vi "Autonomous Independent.vi"() -> ()   [LabVIEW 2012]
doc: "This VI is called when autonomous begins, and will automatically be terminated when autonomous ends. You can carry out timed or sensor driven robot movement independently without needing to return to the caller."
uses:
  Robot Global Data.vi
  <vilib>/Rock Robotics/WPI/RobotDrive/WPI_RobotDriveGetSetRefNum.vi
  <vilib>/Rock Robotics/WPI/Joystick/WPI_JoystickGetSetRefNum.vi
panel:
  in  "Turn Amount":i32=90
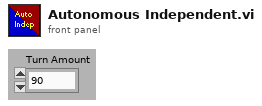
[diagram p1: front panel]
types:
  T1 = typedef "WPI_JoystickDevRef.ctl" = cluster{"Device":T2}
  T2 = typedef "WPI_JoystickDeviceEnum.ctl" = enum16{"USB 1", "USB 2", "USB 3", "USB 4", "Kinect 1", "Kinect 2"}
  T3 = cluster{"axis 1 (x)":dbl, "axis 2 (y)":dbl, "axis 3 (throttle)":dbl, "axis 4":dbl, "axis 5":dbl, "axis 6":dbl}
  T4 = typedef "WPI_RobotDriveDevRef.ctl" = cluster{"DevStatus":errorcluster, "Motors[]":T5[], "Square Inputs":bool, "Max Output":dbl, "Isochronous":bool}
  T5 = typedef "WPI_MotorControlDeviceRef.ctl" = cluster{"DeviceStatus":errorcluster, "Type":enum16{"PWM", "CAN"}, "PWM":cluster{"Digital Module":T6, "PWM Channel":T7, "DeadBand":T8}, "CAN":cluster{"Device Number":u8, "Control Mode":T9, "Semaphore":T10, "Max Vout":dbl}, "Invert":bool, "TransformRef":T11, "InvTransformRef":T11}
  T6 = typedef "FPGA_TypedefDigitalModule.ctl" = enum16{"Digital Module 1", "Digital Module 2"}
  T7 = typedef "FPGA_DIOPWMChannel.ctl" = enum8{"PWM 1", "PWM 2", "PWM 3", "PWM 4", "PWM 5", "PWM 6", "PWM 7", "PWM 8", "PWM 9", "PWM 10", "Invalid"}
  T8 = typedef "WPI_PWMDeadband.ctl" = cluster{"Name":string, "maxPositivePwm":i32, "minPositivePwm":i32, "centerPwm":i32, "maxNegativePwm":i32, "minNegativePwm":i32, "angularRange":u16}
  T9 = typedef "WPI_CANJaguar_ControlMode.ctl" = enum8{"Percent VBus", "Current", "Speed", "Position", "Voltage"}
  T10 = typedef "Semaphore RefNum" = refnum<k1>
  T11 = typedef "WPI_PWMTransform_ConPane.ctl" = refnum<vi>
  T12 = typedef "WPI_GyroDevRef.ctl" = cluster{"DevStatus":errorcluster, "Analog Module":T13, "Analog Channel":T14, "Offset":dbl, "Gain (VoltsPerDegree/Second)":dbl}
  T13 = typedef "FPGA_TypedefAnalogModule.ctl" = enum16{"Analog Module 1", "Analog Module 2"}
  T14 = typedef "FPGA_AIChannel.ctl" = enum8{"AI 1", "AI 2", "AI 3", "AI 4", "AI 5", "AI 6", "AI 7", "AI 8", "Invalid"}
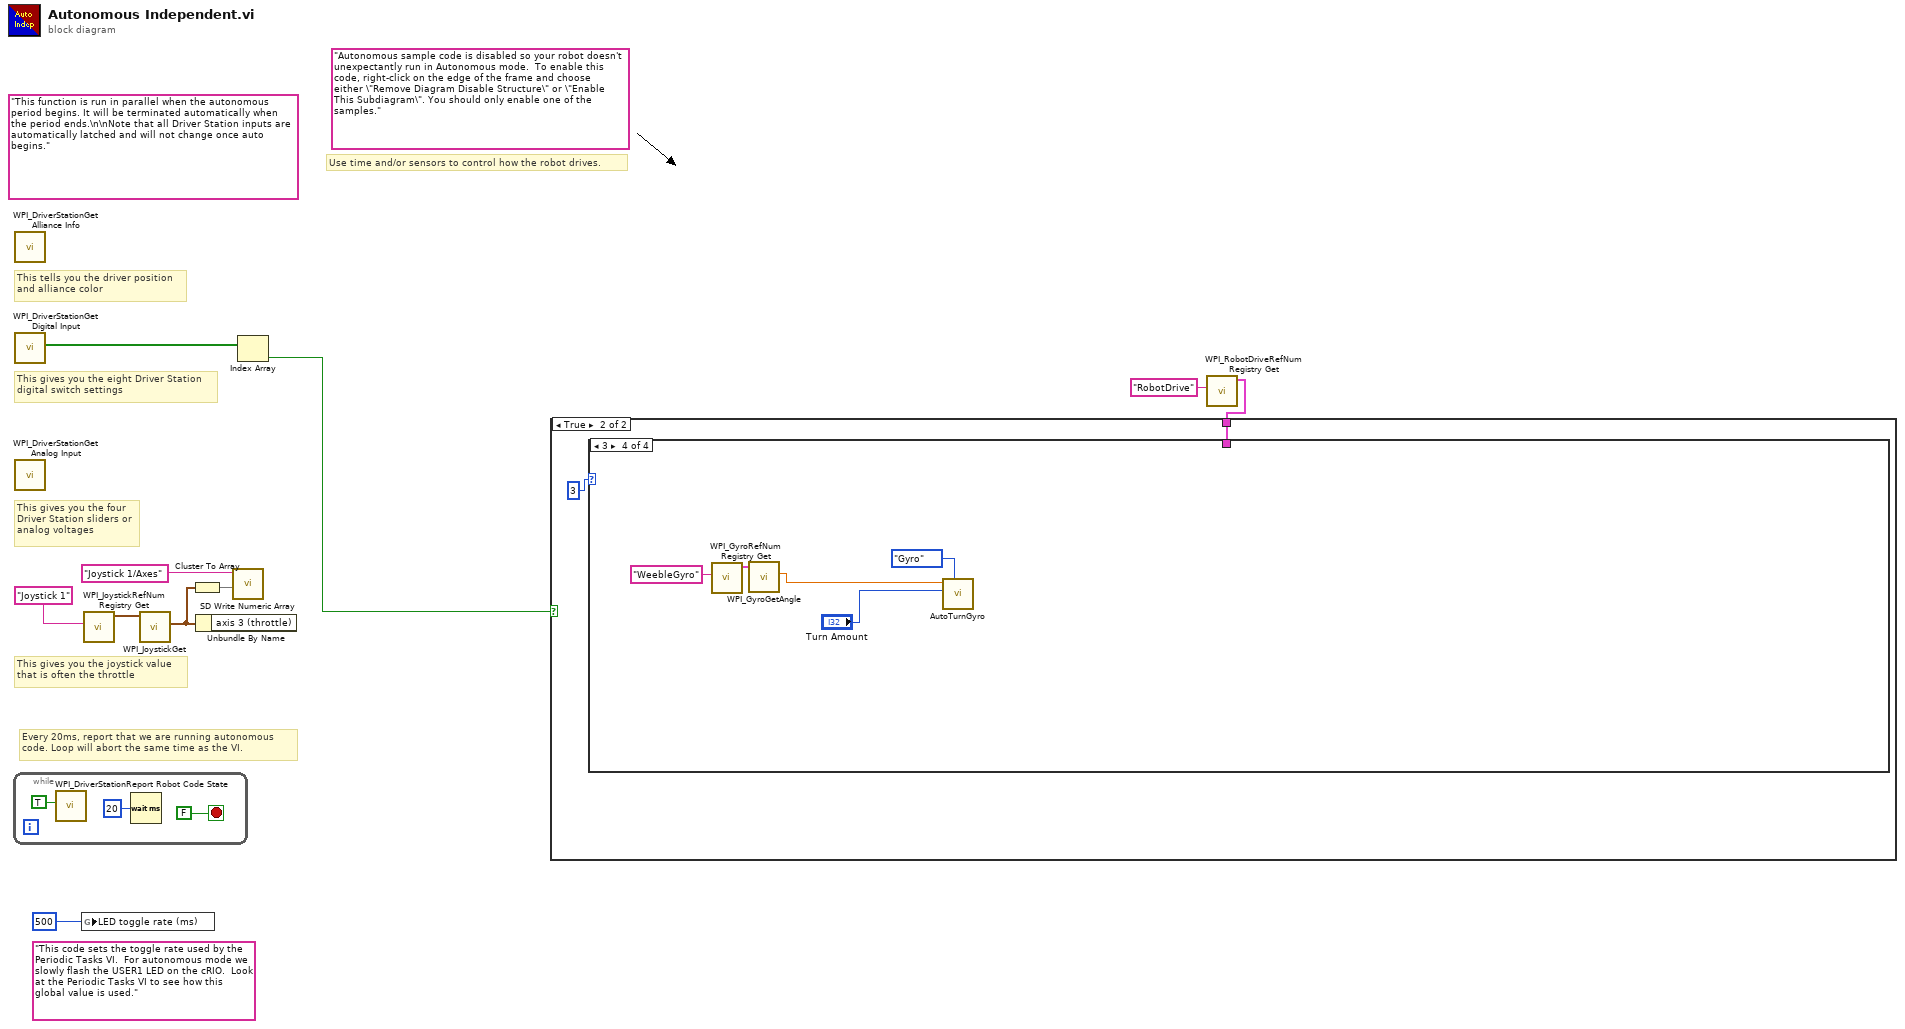
[diagram p0: block diagram]
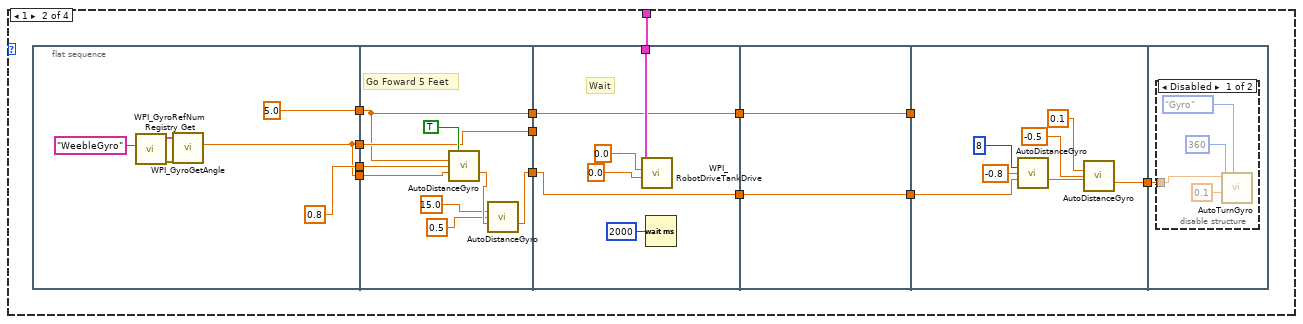
[diagram p4: hidden frame]
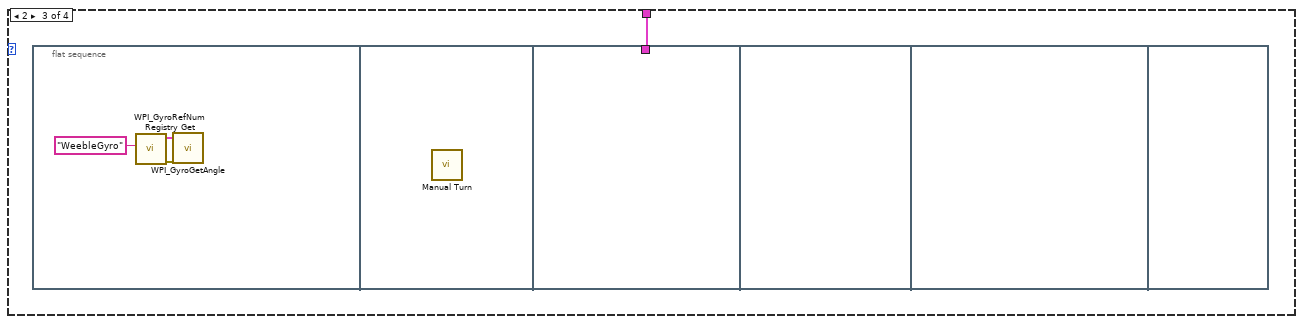
[diagram p6: hidden frame]
diagram:
  (unwired) "This code sets the toggle rate used by the Periodic Tasks VI.  For autonomous mode we slowly flash the USER1 LED on the cRIO.  Look at the Periodic Tasks VI to see how this global value is used."
  (unwired) "Autonomous sample code is disabled so your robot doesn't unexpectantly run in Autonomous mode.  To enable this code, right-click on the edge of the frame and choose either \"Remove Diagram Disable Structure\" or \"Enable This Subdiagram\". You should only enable one of the samples."
  (unwired) "This function is run in parallel when the autonomous period begins. It will be terminated automatically when the period ends.\n\nNote that all Driver Station inputs are automatically latched and will not change once auto begins."
  # "Every 20ms, report that we are running autonomous\ncode. Loop will abort the same time as the VI."
  # "This gives you the joystick value\nthat is often the throttle"
  # "Use time and/or sensors to control how the robot drives."
  # "This tells you the driver position\nand alliance color"
  # "This gives you the eight Driver Station\ndigital switch settings"
  # "This gives you the four\nDriver Station sliders or\nanalog voltages"
  n1 = while {
    stop <- FALSE stop-if-true
    n2 = call <vilib>:"WPI_DriverStationReport Robot Code State.vi"("Autonomous"=TRUE) -> ()  [unwired: 10 in, 1 out]
    n3 = Wait (ms)(milliseconds to wait=u32 20) -> ()  [unwired: 1 out]
  }
  n4 = call <vilib>:"WPI_DriverStationGet Alliance Info.vi"() -> ()  [unwired: 12 out]
  n5 = call <vilib>:"WPI_DriverStationGet Digital Input.vi"() -> ("Driver Station Digital Input (1-8)"=w10:bool[])  [unwired: 11 out]
  n6 = call <vilib>:"WPI_DriverStationGet Analog Input.vi"() -> ()  [unwired: 12 out]
  n7 = global write "Robot Global Data.vi" "LED toggle rate (ms)"(u32 500 ("LED ms toggle rate")) -> ()
  n8 = call <vilib>:"WPI_JoystickRefNum Registry Get.vi"("refnum name"="Joystick 1") -> ("JoystickDevRef"=w8:T1)  [unwired: 1 in, 9 out]
  n9 = call <vilib>:"WPI_JoystickGet.vi"("JoystickDevRef"=w8) -> ("Axes"=w5:T3)  [unwired: 1 in, 5 out]
  n10 = Cluster To Array(cluster=w5) -> (array=w6:dbl[])
  n11 = Unbundle By Name(w5) -> ()  [unwired: 1 out]
  n12 = call <vilib>:"SD Write Numeric Array.vi"("Numeric Array"=w6, "Name"="Joystick 1/Axes") -> ()  [unwired: 8 in, 2 out]
  n13 = Index Array(array=w10) -> (element=w3:bool)  [unwired: 1 in]
  n14 = call <vilib>:"WPI_RobotDriveRefNum Registry Get.vi"("refnum name"="RobotDrive") -> ("RobotDriveDevRef"=w2:T4)  [unwired: 9 in, 1 out]
  n15 = case shown="True" w3 {
    tunnel: w2 -> [_ w15]
    frame False {
    }
    frame True {
      n16 = case shown="3" 3 {
        tunnel: w15 -> [_ w16 w64 _]
        frame 0, Default {
        }
        frame 1 {
          n17 = flat-sequence {
            tunnel: [w29] -> w28
            tunnel: [5.0 ("TargetDistance")] -> w27
            tunnel: [0.8 ("Motor Speed")] -> w26
            tunnel: [w29] -> w25
            tunnel: w28 -> [w42]
            tunnel: w27 -> [w39]
            tunnel: w26 -> [w41]
            tunnel: [w37] -> w24
            tunnel: w25 -> [w40]
            tunnel: [w40] -> w23
            tunnel: [w39] -> w22
            tunnel: w24 -> [w46]
            tunnel: w23 -> [_]
            tunnel: w16 -> [w47]
            tunnel: [w46] -> w21
            tunnel: [w45] -> w20
            tunnel: w22 -> [w45]
            tunnel: [w51] -> w19
            tunnel: w21 -> [w51]
            tunnel: [w50] -> w18
            tunnel: w20 -> [w50]
            tunnel: w19 -> [w58]
            tunnel: w18 -> [_]
            tunnel: [w52] -> w17
            tunnel: w17 -> [w59]
            frame #0 {
              n18 = call <vilib>:"WPI_GyroRefNum Registry Get.vi"("refnum name"="WeebleGyro") -> ("error out"=w34:errorcluster, "GyroDevRef"=w33:T12)  [unwired: 9 in]
              n19 = call <vilib>:"WPI_GyroGetAngle.vi"("error in (no error)"=w34, "GyroDevRef"=w33) -> ("Angle"=w29:dbl)  [unwired: 6 in, 3 out]
            }
            frame #1 {
              # "Go Foward 5 Feet"
              n20 = call "AutoDistanceGyro.vi"("Reset Encoders"=TRUE, "TargetDistance"=w39, "Motor Speed"=w41, "InitialAngle"=w42) -> ("InitialAngle Out"=w38:dbl)  [unwired: 10 in, 1 out]
              n21 = call "AutoDistanceGyro.vi"("TargetDistance"=15.0, "Motor Speed"=0.5, "InitialAngle"=w38) -> ("InitialAngle Out"=w37:dbl)  [unwired: 11 in, 1 out]
            }
            frame #2 {
              # "Wait"
              n22 = call <vilib>:"WPI_RobotDriveTankDrive.vi"("Right axis value"=0.0 ("Y axis value"), "Left axis value"=0.0 ("X axis value"), "RobotDriveDevRef"=w47) -> ()  [unwired: 6 in, 3 out]
              n23 = Wait (ms)(milliseconds to wait=u32 2000) -> ()  [unwired: 1 out]
            }
            frame #3 {
            }
            frame #4 {
              n24 = call "AutoDistanceGyro.vi"("TargetDistance"=8, "Motor Speed"=-0.8, "InitialAngle"=w58) -> ("InitialAngle Out"=w55:dbl)  [unwired: 11 in, 1 out]
              n25 = call "AutoDistanceGyro.vi"("TargetDistance"=0.1, "Motor Speed"=-0.5, "InitialAngle"=w55) -> ("InitialAngle Out"=w52:dbl)  [unwired: 11 in, 1 out]
            }
            frame #5 {
              n26 = disable-structure shown="Disabled" {
                disable-tunnel: w59 -> [w61 _]
                frame Disabled {
                  n27 = call "AutoTurnGyro.vi"("Sensor (Gyro)"=enum16{"Gyro", "Vision"}."Gyro", 9:0.1 ("Error Tolerence"), "Turn Amount"=360, "Initial Angle"=w61) -> ()  [unwired: 6 in, 2 out]
                }
                frame Enabled {
                }
              }
            }
          }
        }
        frame 2 {
          n28 = flat-sequence {
            tunnel: w64 -> [_]
            frame #0 {
              n29 = call <vilib>:"WPI_GyroRefNum Registry Get.vi"("refnum name"="WeebleGyro") -> ("error out"=w67:errorcluster, "GyroDevRef"=w66:T12)  [unwired: 9 in]
              n30 = call <vilib>:"WPI_GyroGetAngle.vi"("error in (no error)"=w67, "GyroDevRef"=w66) -> ()  [unwired: 6 in, 4 out]
            }
            frame #1 {
              n31 = call "Manual Turn.vi"() -> ()  [unwired: 12 in]
            }
            frame #2 {
            }
            frame #3 {
            }
            frame #4 {
            }
            frame #5 {
            }
          }
        }
        frame 3 {
          n32 = call <vilib>:"WPI_GyroRefNum Registry Get.vi"("refnum name"="WeebleGyro") -> ("GyroDevRef"=w70:T12)  [unwired: 9 in, 1 out]
          n33 = call <vilib>:"WPI_GyroGetAngle.vi"("GyroDevRef"=w70) -> ("Angle"=w68:dbl)  [unwired: 7 in, 3 out]
          n34 = call "AutoTurnGyro.vi"("Sensor (Gyro)"=enum16{"Gyro", "Vision"}."Gyro", "Turn Amount"="Turn Amount", "Initial Angle"=w68) -> ()  [unwired: 7 in, 2 out]
        }
      }
    }
  }
